vi "from_item.vi"(8 "error in (no error)":errorcluster, 10 "item_ref":u64) -> (0 "error out":errorcluster, 3 "Table out":refnum<class "InlineTable.lvclass">)   [LabVIEW 2020, in "toml_edit.lvlib" / "InlineTable.lvclass"]
uses:
  InlineTable.lvclass
  InlineTable.lvclass/InlineTable.ctl
  dragon_toml_64.dll
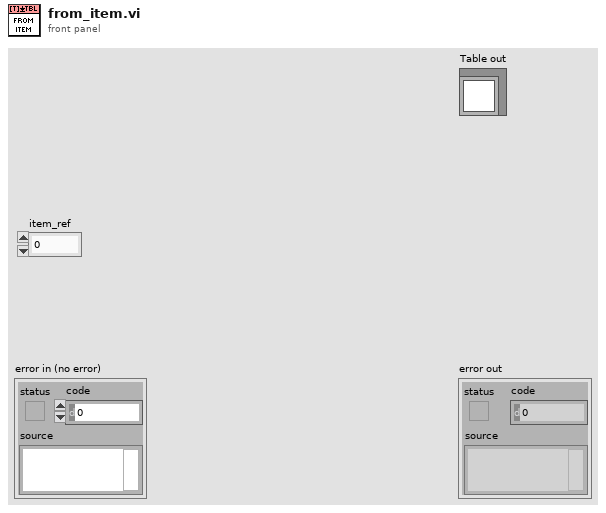
[diagram p1: front panel]
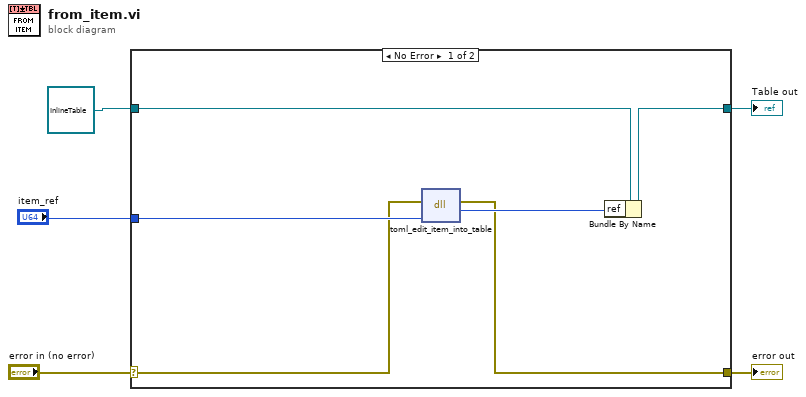
[diagram p0: block diagram]
diagram:
  n1 = case shown="No Error" "error in (no error)" {
    selector: "error in (no error)" -> [w9 w13]
    tunnel: [w8 w13] -> w4
    tunnel: [w7 w12] -> w2
    tunnel: refnum<class "InlineTable.lvclass"> refnum ("Table in") -> [w6 w12]
    tunnel: "item_ref" -> [w10 _]
    frame No Error {
      n2 = dll-call lib="C:/Projects/toml-edit-labview/lv_src/dragon_toml_*.dll" fn="toml_edit_item_into_table"(error in=w9, "item"=w10) -> (error out=w8:errorcluster, "table"=w11:u64)  [unwired: 3 in, 1 out]
      n3 = Bundle By Name(cluster=w6, "ref"=w11) -> (w7:refnum<class "InlineTable.lvclass">)
    }
    frame Error {
    }
  }
  "error out" <- w4
  "Table out" <- w2
